vi "unbuffered_intensity_graph.vi"() -> ()   [LabVIEW 2019]
panel:
  in  "stop":bool
  out "Intensity Graph":dbl[][](graph)
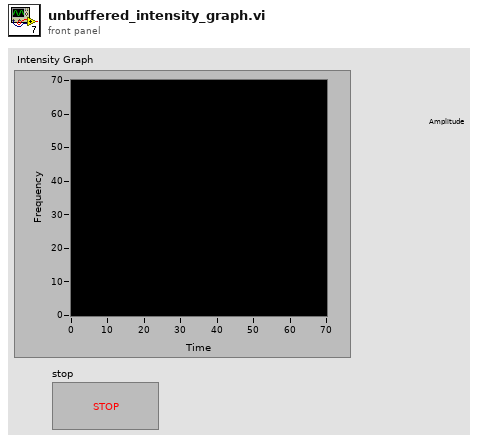
[diagram p1: front panel]
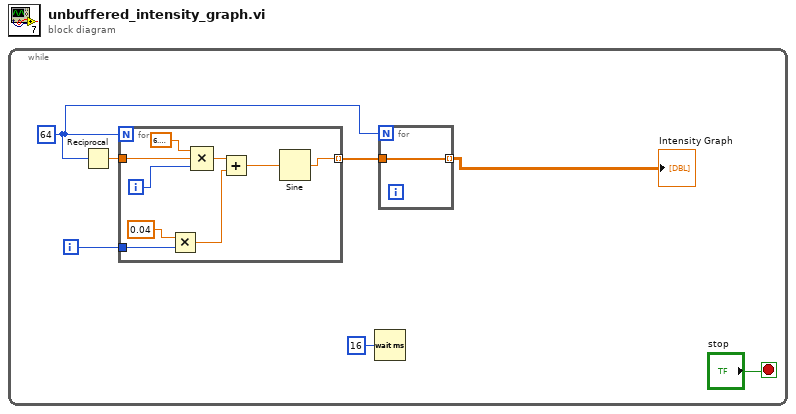
[diagram p0: block diagram]
diagram:
  n1 = while {
    i -> [w3]
    stop <- "stop" stop-if-true
    w4 = 64
    n2 = Reciprocal(x=w4) -> (1/x=w6:dbl)
    n3 = for {
      N: w4 -> [_]
      tunnel: w6 -> [w16]
      tunnel: [w9] -> w5 mode=indexing
      tunnel: w3 -> [w14]
      i -> [w15]
      n4 = Multiply(x=0.04, y=w14) -> (x*y=w11:dbl)
      n5 = Compound Arithmetic op=MULTIPLY(6.283185307179586, w16, w15) -> (w12:dbl)
      n6 = Add(x=w12, y=w11) -> (x+y=w10:dbl)
      n7 = Sine(x=w10) -> (sin(x)=w9:dbl)
    }
    n8 = Wait (ms)(milliseconds to wait=u32 16) -> ()  [unwired: 1 out]
    n9 = for {
      N: w4 -> [_]
      tunnel: w5 -> [w8]
      tunnel: [w8] -> w2 mode=indexing
    }
    "Intensity Graph" <- w2
  }
